vi "reference and uncalibrated.vi"(4 "Reference Index":u32, 5 "uncalibrated index":u32, 7 "scaled data":sgl[][](array[numeric]) format="%.5f") -> (3 "reference and volts":sgl[][](array[numeric]) format="%.5f")   [LabVIEW 2015]
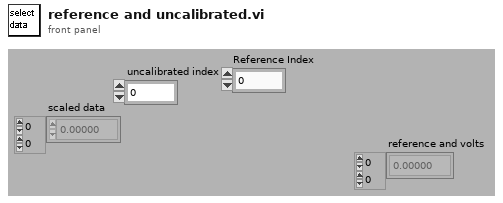
[diagram p1: front panel]
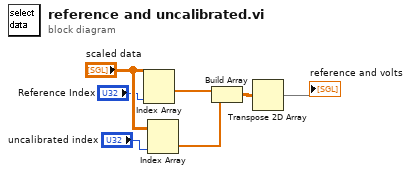
[diagram p0: block diagram]
diagram:
  n1 = Index Array(array="scaled data", index (col)="Reference Index") -> (element=w6:sgl[])  [unwired: 1 in]
  n2 = Index Array(array="scaled data", index (col)="uncalibrated index") -> (element=w5:sgl[])  [unwired: 1 in]
  n3 = Build Array(w6, w5) -> (w4:sgl[][])
  n4 = Transpose 2D Array(2D array=w4) -> (transposed array=→"reference and volts":sgl[][])
